vi "myRIO_BRig_Host_formatData_getHeaders_dataMTrig.vi"() -> (3 "output_stringArray_dataMTrig":string[](array[string]))   [LabVIEW 2014]
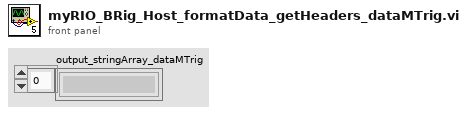
[diagram p1: front panel]
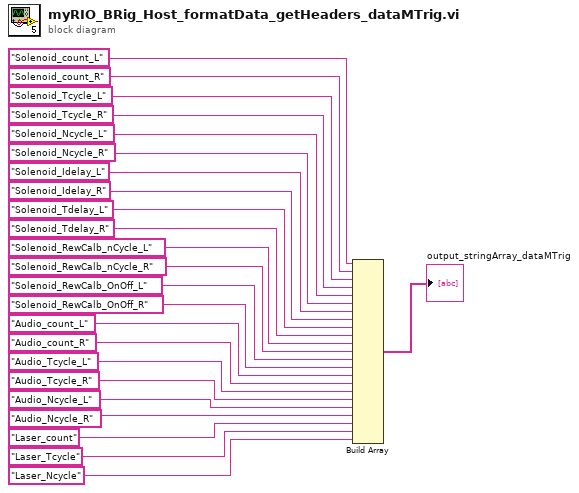
[diagram p0: block diagram]
diagram:
  n1 = Build Array("Solenoid_count_L", "Solenoid_count_R", "Solenoid_Tcycle_L", "Solenoid_Tcycle_R", "Solenoid_Ncycle_L", "Solenoid_Ncycle_R", "Solenoid_Idelay_L", "Solenoid_Idelay_R", "Solenoid_Tdelay_L", "Solenoid_Tdelay_R", "Solenoid_RewCalb_nCycle_L", "Solenoid_RewCalb_nCycle_R", "Solenoid_RewCalb_OnOff_L", "Solenoid_RewCalb_OnOff_R", "Audio_count_L", "Audio_count_R", "Audio_Tcycle_L", "Audio_Tcycle_R", "Audio_Ncycle_L", "Audio_Ncycle_R", "Laser_count", "Laser_Tcycle", "Laser_Ncycle") -> (→"output_stringArray_dataMTrig":string[])
